vi "Initialize Dependencies Attribute.vi"() -> (3 "Attribute.Dependencies":refnum<class "Attribute.Dependencies.lvclass">)   [LabVIEW 2021, in "smo.lvlib" / "Attribute.Dependencies.lvclass"]
uses:
  Attribute.Dependencies.lvclass
  C:/Repositories/SMO/src/Support/Attribute/Attribute.lvclass
  Definitions/def.SMO/Scope -- Enum.ctl
  Attribute/Attribute.lvclass/Attribute.ctl
  Attribute.Dependencies.lvclass/Attribute.Dependencies.ctl
  Definitions/def.SMO/def.SMO.lvclass
  Attribute/Attribute.lvclass
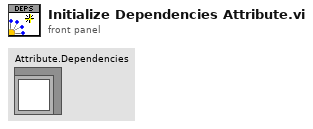
[diagram p1: front panel]
types:
  T1 = typedef "smo.lvlib/def.SMO.lvclass/Scope -- Enum.ctl" = enum16{"Public", "Protected", "Private"}
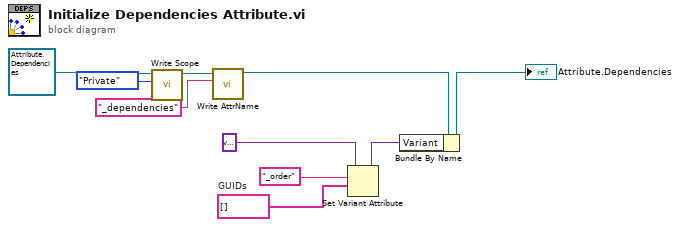
[diagram p0: block diagram]
diagram:
  w6 = string[] []  # GUIDs
  n1 = call "Write Scope.vi"("Scope"=Scope_--_Enum."Private", "Attribute in"=refnum<class "Attribute.Dependencies.lvclass"> refnum ("Attribute.Owner in")) -> ("Attribute out"=w3:refnum<class "Attribute.Dependencies.lvclass">)  [unwired: 9 in]
  n2 = call "Write AttrName.vi"("Attribute Name"="_dependencies", "Attribute in"=w3) -> ("Attribute in"=w1:refnum<class "Attribute.Dependencies.lvclass">)  [unwired: 9 in]
  n3 = Set Variant Attribute(Variant=variant, name="_order" ("Attribute Name"), value=w6) -> (Variant out=w8:variant)  [unwired: 1 in, 2 out]
  n4 = Bundle By Name(cluster=w1, "Variant"=w8) -> (→"Attribute.Dependencies":refnum<class "Attribute.Dependencies.lvclass">)
